vi "LWXPS_CIERegister64ValueGet.vi"(0 "XPS Reference IN":refnum<k24>, 5 "Positioner Name":string, 7 "Board Offset":i16, 11 "LabVIEW error IN":errorcluster) -> (4 "XPS Reference OUT":refnum<k24>, 6 "Returned error code":i32, 8 "Register Value":i32, 10 "XPS Error String":string, 15 "LabVIEW error OUT":errorcluster)   [LabVIEW 2014]
uses:
  D:/XPSQ8_LabView_Library/Development/Source/Dll/Newport.XPS.CommandInterface.dll
  Dll/Newport.XPS.CommandInterface.dll
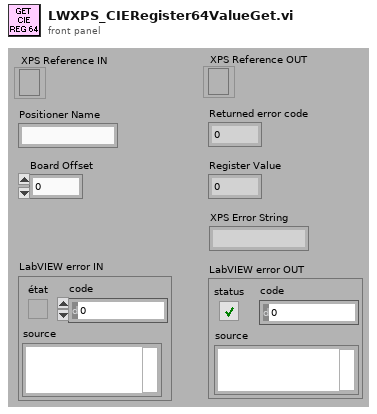
[diagram p1: front panel]
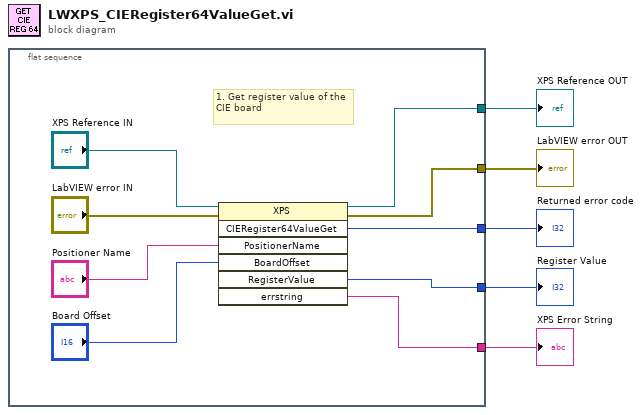
[diagram p0: block diagram]
diagram:
  n1 = flat-sequence {
    tunnel: [w12] -> w5
    tunnel: [w11] -> w4
    tunnel: [w7] -> w3
    tunnel: [w10] -> w2
    tunnel: [w6] -> w1
    frame #0 {
      # "1. Get register value of the CIE board"
      n2 = invoke class="XPS" method="CIERegister64ValueGet"(reference="XPS Reference IN", error in="LabVIEW error IN", "PositionerName"="Positioner Name", "BoardOffset"="Board Offset") -> (reference out=w12:refnum<k24>, error out=w11:errorcluster, "CIERegister64ValueGet"=w6:i32, "RegisterValue"=w10:i32, "errstring"=w7:string)  [unwired: 3 in, 2 out]
    }
  }
  "XPS Reference OUT" <- w5
  "LabVIEW error OUT" <- w4
  "XPS Error String" <- w3
  "Register Value" <- w2
  "Returned error code" <- w1
